vi "Get reading.vi"(8 "error in (no error)":errorcluster, 10 "Frequency (GHz)":dbl, 11 "Power control in":refnum<class "Power control.lvclass">) -> (0 "error out":errorcluster, 2 "Power (mW)":dbl, 3 "Power control out":refnum<class "Power control.lvclass">)   [LabVIEW 2015, in "Power control.lvclass"]
uses:
  Power control.lvclass
  Power control.lvclass/Power control.ctl
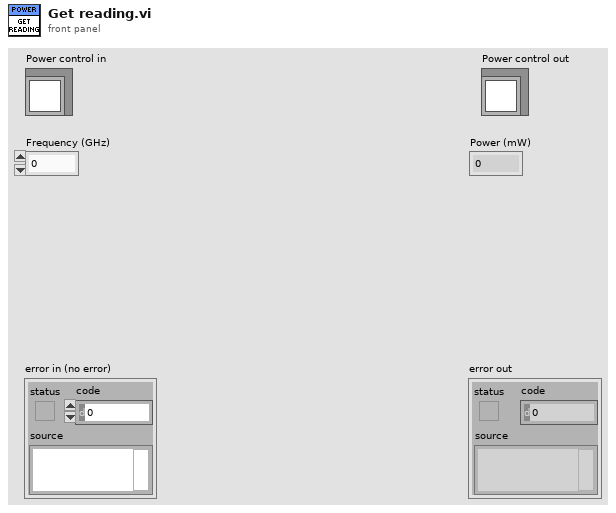
[diagram p1: front panel]
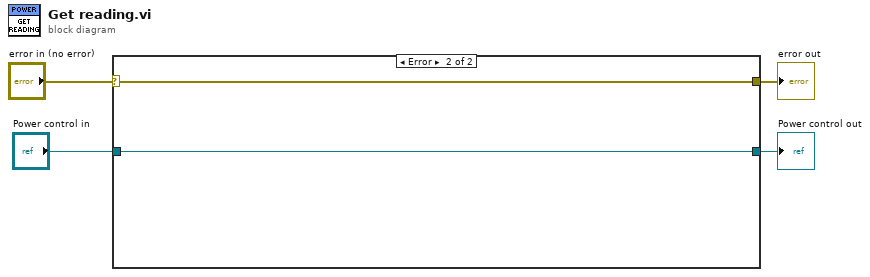
[diagram p0: block diagram]
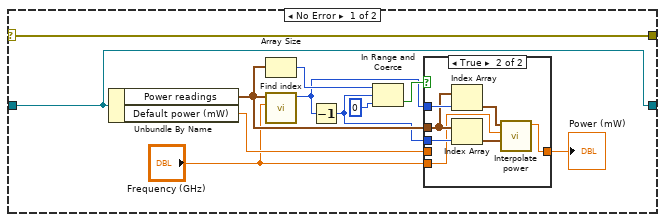
[diagram p2: hidden frame]
diagram:
  n1 = case shown="Error" "error in (no error)" {
    selector: "error in (no error)" -> [w15 w25]
    tunnel: [w15 w25] -> w3
    tunnel: "Power control in" -> [w5 w24]
    tunnel: [w5 w24] -> w1
    frame No Error {
      n2 = Unbundle By Name(w5) -> ("Power readings"=w9:cluster{"Frequency":dbl, "Power":dbl}[], "Default power (mW)"=w11:dbl)
      n3 = Array Size(array=w9) -> (size(s)=w14:i32)
      n4 = call "Find index.vi"("Frequency (GHz)"="Frequency (GHz)", "Power readings"=w9) -> ("Index of matching or greater point"=w7:i32)  [unwired: 9 in]
      n5 = Decrement(x=w7) -> (x-1=w8:i32)
      n6 = In Range and Coerce(upper limit=w14, x=w8, lower limit=0) -> (In Range?=w12:bool)  [unwired: 1 out]
      n7 = case shown="True" w12 {
        tunnel: w11 -> [w16 _]
        tunnel: [w16 w18] -> w10
        tunnel: w9 -> [_ w21]
        tunnel: w8 -> [_ w23]
        tunnel: w7 -> [_ w22]
        tunnel: "Frequency (GHz)" -> [_ w17]
        frame False {
        }
        frame True {
          n8 = Index Array(array=w21, index=w22) -> (element=w20:cluster{"Frequency":dbl, "Power":dbl})
          n9 = Index Array(array=w21, index=w23) -> (element=w19:cluster{"Frequency":dbl, "Power":dbl})
          n10 = call "Interpolate power.vi"("Point below"=w19, "Frequency (GHz)"=w17, "Point above"=w20) -> ("Power (mW)"=w18:dbl)  [unwired: 8 in]
        }
      }
      "Power (mW)" <- w10
    }
    frame Error {
    }
  }
  "error out" <- w3
  "Power control out" <- w1
